vi "Read Data and Search for Property Value.vi"() -> ()   [LabVIEW 2014]
uses:
  <vilib>/Utility/file.llb/Read From Spreadsheet File (string).vi
panel:
  in  "Property Name":string="UUT Serial Number"
  out "Property Value":string
  out "Spreadsheet file in array form":string[][](array[string])
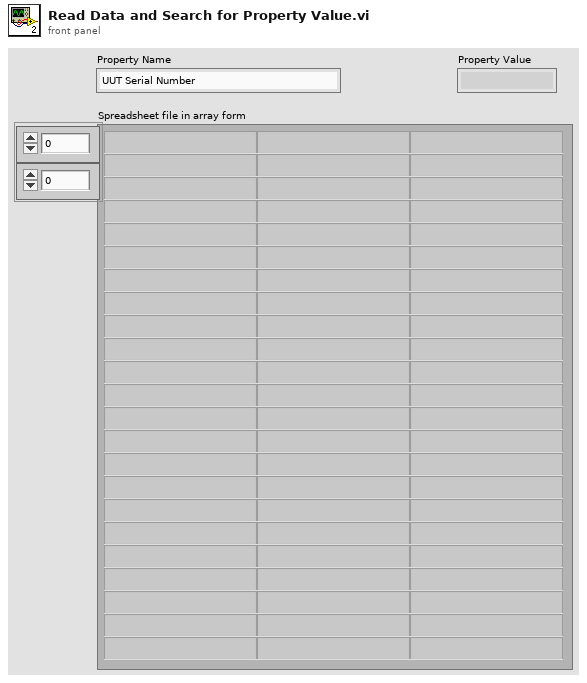
[diagram p1: front panel]
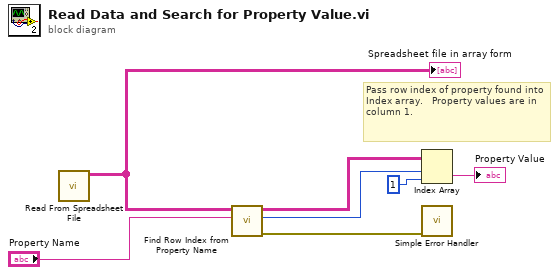
[diagram p0: block diagram]
diagram:
  # "Pass row index of property found into Index array.   Property values are in column 1."
  n1 = call-poly <vilib>:"Read From Spreadsheet File.vi"() -> ("all rows"=w7:string[][])  [unwired: 7 in, 4 out]
  "Spreadsheet file in array form" <- w7
  n2 = call "Find Row Index from Property Name.vi"("Property Name"="Property Name", "Spreadsheet String Array"=w7) -> ("Error Out"=w1:errorcluster, "Row Index"=w6:i32, "Spreadsheet String Array Out"=w5:string[][])  [unwired: 7 in]
  n3 = Index Array(array=w5, index (row)=w6, index (col)=1 ("length")) -> (element=→"Property Value":string)
  n4 = call <vilib>:"Simple Error Handler.vi"("error in (no error)"=w1) -> ()  [unwired: 4 in, 5 out]
